vi "LastSample_171213.vi"(8 "BufferLengthSamples":u32=10000, 10 "InputArray":sgl[][](array[numeric]), 11 "i":u32=10000) -> (3 "OutputArray":sgl[][](array[numeric]))   [LabVIEW 2016]
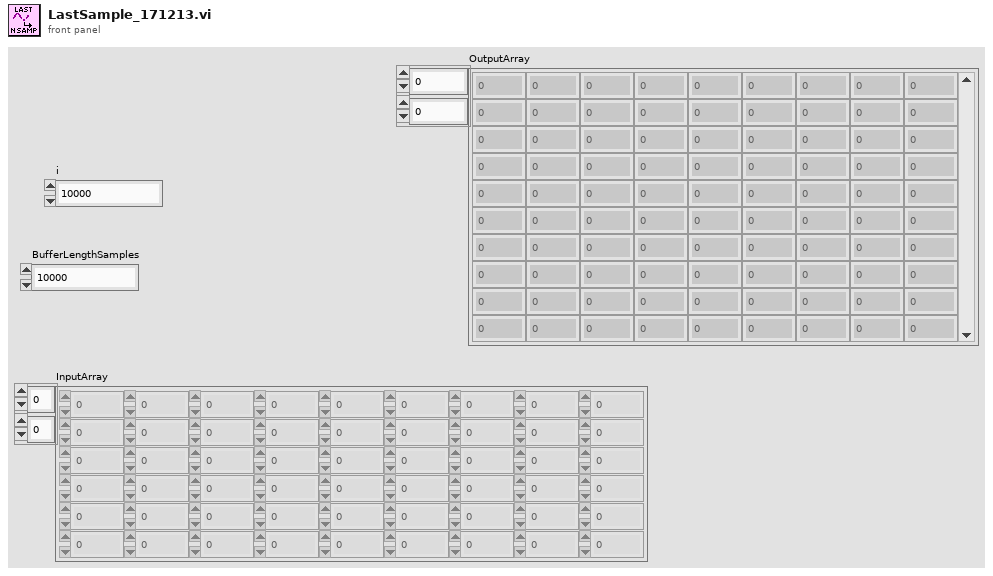
[diagram p1: front panel]
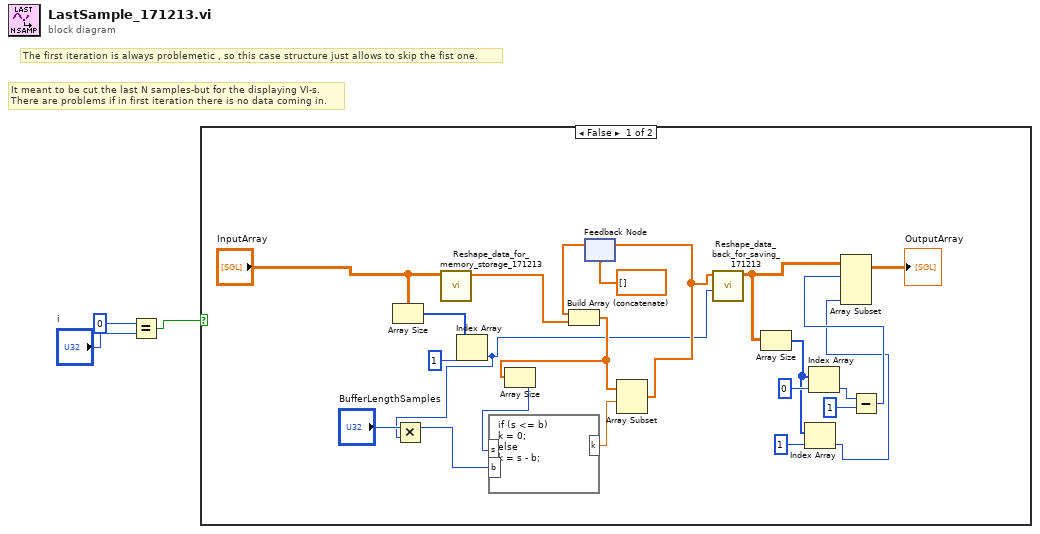
[diagram p0: block diagram]
diagram:
  # "It meant to be cut the last N samples-but for the displaying VI-s.\nThere are problems if in first iteration there is no data coming in."
  # "The first iteration is always problemetic , so this case structure just allows to skip the fist one."
  n1 = Equal?(x=u32 0, y="i") -> (x = y?=w1:bool)
  n2 = case shown="False" w1 {
    frame False {
      n3 = Array Size(array="InputArray") -> (size(s)=w9:i32[])
      n4 = call "Reshape_data_for_memory_storage_171213.vi"("DEC SGL input"="InputArray") -> ("DEC SGL Output"=w17:sgl[])  [unwired: 10 in]
      n5 = Index Array(array=w9, index=1) -> (element=w6:i32)
      n6 = Multiply(x="BufferLengthSamples", y=w6) -> (x*y=w7:u32)
      n7 = feedback #1(sgl[] []) -> (w16:sgl[])
      n8 = Build Array (concatenate)(w16, w17) -> (w14:sgl[])
      n9 = Array Size(array=w14) -> (size(s)=w13:i32)
      n10 = formula code="if (s <= b)\nk = 0;\nelse\nk = s - b;"("s"=w13, "b"=w7) -> ("k"=w12:dbl)
      n11 = Array Subset(array=w14, index=w12) -> (w15:sgl[])  [unwired: 1 in]
      n12 = feedback-in #1(w15) -> ()
      n13 = call "Reshape_data_back_for_saving_171213.vi"("Read frame size"=w6, "DEC SGL input"=w15) -> ("DEC SGL Output"=w21:sgl[][])  [unwired: 9 in]
      n14 = Array Size(array=w21) -> (size(s)=w20:i32[])
      n15 = Index Array(array=w20, index=1) -> (element=w5:i32)
      n16 = Index Array(array=w20, index=0) -> (element=w23:i32)
      n17 = Subtract(x=w23, y=1) -> (x-y=w19:i32)
      n18 = Array Subset(array=w21, index (row)=w19, length (col)=w5) -> (→"OutputArray":sgl[][])  [unwired: 2 in]
    }
    frame True {
    }
  }
